vi "Grid_Main.vi"(9 "DC images in":dbl[][][](array[numeric]), 10 "Part of multigrid":bool, 11 "Settings":T3={"Drift Correction Settings"={"Drift Correction every"=1, "Drift correction Pixels"=256, "Channel index (0-23)"=0, "MaxImagesBack"=2, "Threshold"=2, "Increment"=1, "max applied Drift Correction"=20, "Correct Drift"=TRUE, "Correlate"=0, "Correct z drift"=FALSE, "zdrift \nDuration (s)"=0.0}, "Spectroscopy Setting"={"Imaging Current"=5e-12, "ref Current"=5e-12, "tip Speed (m/s)"=2e-09, "Imaging Bias"=0.02, "ref Bias"=0.02, "preSTS delay [ms]"=2000, "STS z offset"=0.0, "during Spec Bias (V)"=0.0015, "trigger1 < Hz"=-6.0, "trigger 2 >Hz"=-4.0, "autoStop"=TRUE, "Spectroscopy"=1, "PLL ON/OFF"=TRUE, "readjust setpoint every "=1, "z Reference (constHeight)"=TRUE, "Lock In"=FALSE}, "Misc"={"File name"="MgPc_perturbed_linezSpec1", "Email when finished"="marina.castelli@monash.edu"}, "Grid Settings"={"type"=0, "type order"=0, "X pixel"=20, "Y pixel"=1, "Grid_Parms"={"center X (m)"=-1.7352741e-07, "center Y (m)"=-2.3765438e-07, "width (m)"=-1.740481e-07, "height (m)"=-2.3958808e-07, "angle (deg)"=-1.0}}} {"Grid Settings"."type order" items=["Grid", "Random", "Adam7"]; "Grid Settings"."type" items=["Line", "Grid", "Cloud"]; "Spectroscopy Setting"."Spectroscopy" items=["Bias", "zSpec"]; "Spectroscopy Setting"."trigger 2 >Hz" format="%#_6p"; "Spectroscopy Setting"."trigger1 < Hz" format="%#_6p"; "Spectroscopy Setting"."during Spec Bias (V)" format="%#_5p"; "Spectroscopy Setting"."STS z offset" format="%#_6p"; "Spectroscopy Setting"."ref Bias" format="%#_6p"; "Spectroscopy Setting"."Imaging Bias" format="%#_6p"; "Spectroscopy Setting"."tip Speed (m/s)" format="%.2p"; "Spectroscopy Setting"."ref Current" format="%#_6p"; "Spectroscopy Setting"."Imaging Current" format="%#_6p"; "Drift Correction Settings"."Correlate" items=["first Frame", "successive Frames"]; "Drift Correction Settings"."max applied Drift Correction" min=1 max=100 step=1 format="%.0p"; "Drift Correction Settings"."Threshold" min=1 step=1; "Drift Correction Settings"."Channel index (0-23)" items=["Current"=0, "Z (m)"=14]}) -> (1 "DC images out":dbl[][][](array[numeric]), 3 "Settings out":T2)   [LabVIEW 2014]
uses:
  <userlib>/Nanonis Prog Interface V5/Nanonis Prog Interface.lvlib
panel:
  in  "resume":T1
  in  "stop":bool
  out "total points":i32=20
  out "Points taken":i32=3
  out "ETA":timestamp=timestamp(3632272774.4134703 s since 1904-01-01)
  out "remaining time":dbl=712.12539879481 format="%<%H:%M:%S>t"
  out "Progress":u8(slide)=15 scale=0.0..100.0 scale format="%#.1g"
  out "Last z adjustment":dbl
  out "Last Drift detected (images back)":i32=1
  out "Y Offset out":sgl=-2.34375e-11 format="%#_6p"
  out "X Offset out":sgl format="%#_6p"
  out "Drift Correction Image":picture
  # "RUN smart tilt before starting the GRID\nCHECK CUTOFF\nmove tip to reference point for tip height"
  # "%"
  # "finish the last action and then"
  # "GRID points"
  # "Increase this if no Drift was detected for \na certain number of images"
  # "% of image size"
  # "Only first frame works"
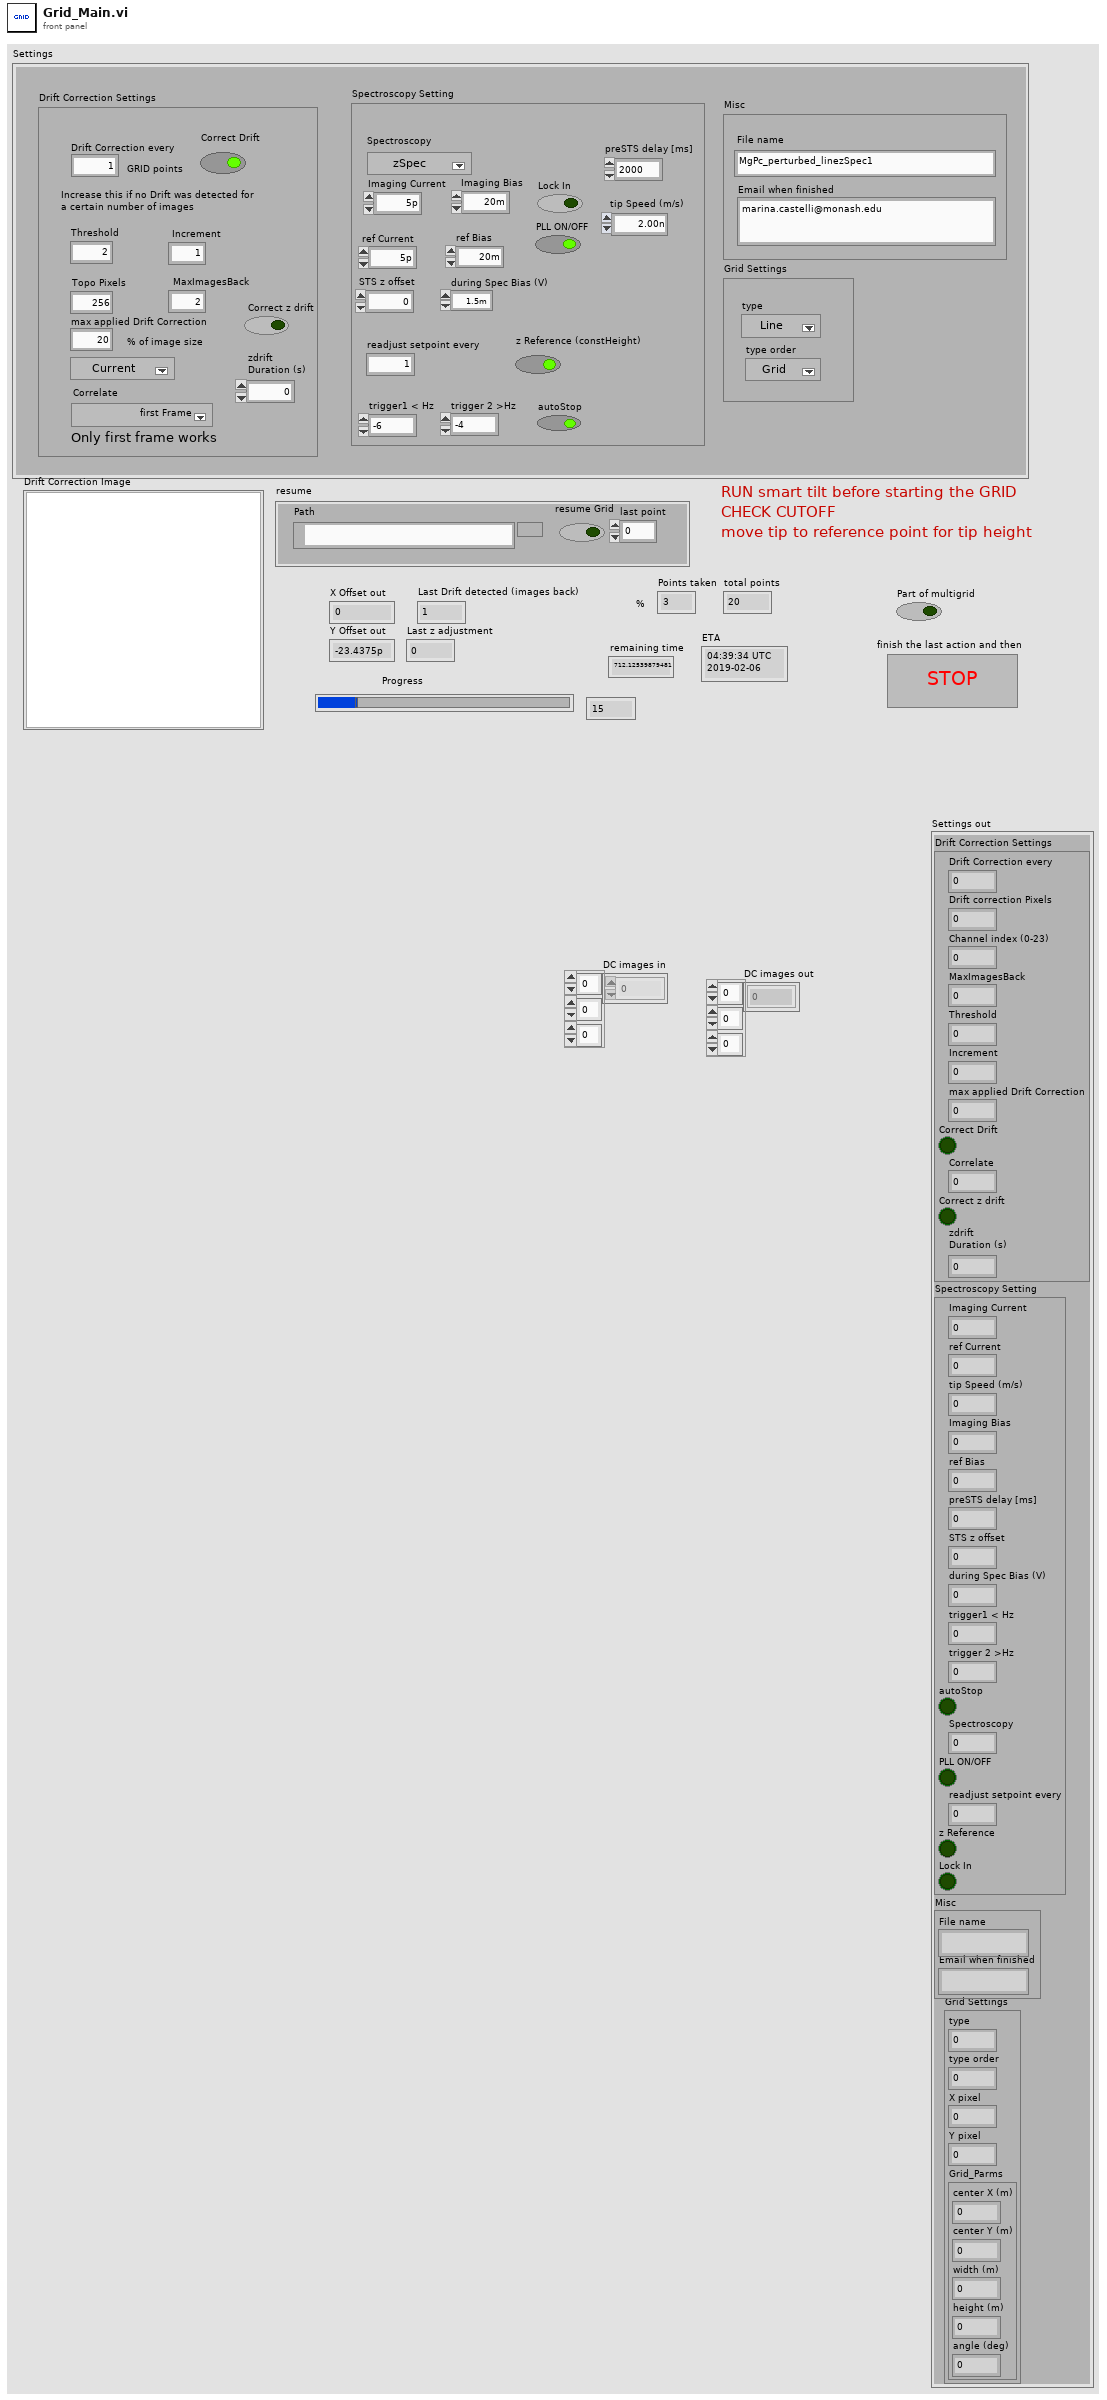
[diagram p1: front panel]
types:
  T1 = cluster{"resume Grid":bool, "Path":path, "last point":i32}
  T2 = cluster{"Drift Correction Settings":cluster{"Drift Correction every":i32, "Drift correction Pixels":i32, "Channel index (0-23)":u8, "MaxImagesBack":i32, "Threshold":i32, "Increment":i32, "max applied Drift Correction":i32, "Correct Drift":bool, "Correlate":u16, "Correct z drift":bool, "zdrift \nDuration (s)":dbl}, "Spectroscopy Setting":cluster{"Imaging Current":dbl, "ref Current":dbl, "tip Speed (m/s)":sgl, "Imaging Bias":dbl, "ref Bias":dbl, "preSTS delay [ms]":u32, "STS z offset":dbl, "during Spec Bias (V)":sgl, "trigger1 < Hz":sgl, "trigger 2 >Hz":sgl, "autoStop":bool, "Spectroscopy":u16, "PLL ON/OFF":bool, "readjust setpoint every ":i32, "z Reference":bool, "Lock In":bool}, "Misc":cluster{"File name":string, "Email when finished":string}, "Grid Settings":cluster{"type":u16, "type order":u16, "X pixel":i32, "Y pixel":i32, "Grid_Parms":cluster{"center X (m)":sgl, "center Y (m)":sgl, "width (m)":sgl, "height (m)":sgl, "angle (deg)":sgl}}}
  T3 = cluster{"Drift Correction Settings":cluster{"Drift Correction every":i32, "Drift correction Pixels":i32, "Channel index (0-23)":u8, "MaxImagesBack":i32, "Threshold":i32, "Increment":i32, "max applied Drift Correction":i32, "Correct Drift":bool, "Correlate":u16, "Correct z drift":bool, "zdrift \nDuration (s)":dbl}, "Spectroscopy Setting":cluster{"Imaging Current":dbl, "ref Current":dbl, "tip Speed (m/s)":sgl, "Imaging Bias":dbl, "ref Bias":dbl, "preSTS delay [ms]":u32, "STS z offset":dbl, "during Spec Bias (V)":sgl, "trigger1 < Hz":sgl, "trigger 2 >Hz":sgl, "autoStop":bool, "Spectroscopy":u16, "PLL ON/OFF":bool, "readjust setpoint every ":i32, "z Reference (constHeight)":bool, "Lock In":bool}, "Misc":cluster{"File name":string, "Email when finished":string}, "Grid Settings":cluster{"type":u16, "type order":u16, "X pixel":i32, "Y pixel":i32, "Grid_Parms":cluster{"center X (m)":sgl, "center Y (m)":sgl, "width (m)":sgl, "height (m)":sgl, "angle (deg)":sgl}}}
  T4 = cluster{"Drift File out":refnum<file>, "zFile":refnum<file>, "BinFile ref":refnum<file>, "xyFile":refnum<file>}
  T5 = cluster{"Drift Correction every":i32, "Drift correction Pixels":i32, "Channel index (0-23)":u8, "MaxImagesBack":i32, "Threshold":i32, "Increment":i32, "max applied Drift Correction":i32, "Correct Drift":bool, "Correlate":u16, "Correct z drift":bool, "zdrift \nDuration (s)":dbl}
  T6 = cluster{"Imaging Current":dbl, "ref Current":dbl, "tip Speed (m/s)":sgl, "Imaging Bias":dbl, "ref Bias":dbl, "preSTS delay [ms]":u32, "STS z offset":dbl, "during Spec Bias (V)":sgl, "trigger1 < Hz":sgl, "trigger 2 >Hz":sgl, "autoStop":bool, "Spectroscopy":u16, "PLL ON/OFF":bool, "readjust setpoint every ":i32, "z Reference":bool, "Lock In":bool}
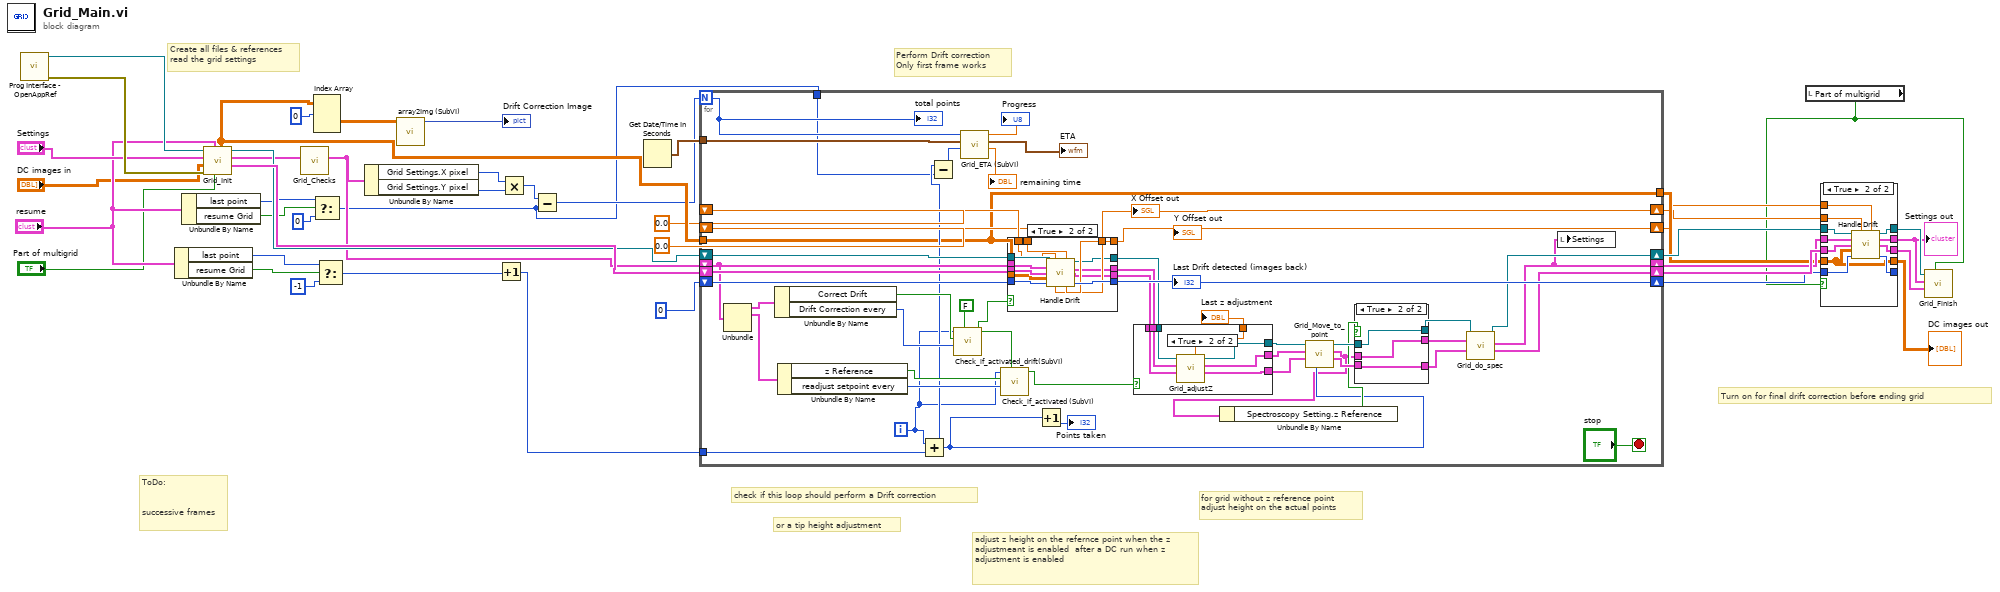
[diagram p0: block diagram]
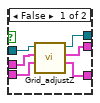
[diagram p3: hidden frame]
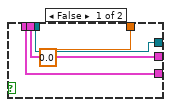
[diagram p4: hidden frame]
diagram:
  # "Turn on for final drift correction before ending grid"
  # "ToDo:\n\n\nsuccessive frames"
  # "Perform Drift correction\nOnly first frame works"
  # "check if this loop should perform a Drift correction"
  # "for grid without z reference point \nadjust height on the actual points"
  # "or a tip height adjustment"
  # "Create all files & references\nread the grid settings"
  # "adjust z height on the refernce point when the z adjustmeant is enabled  after a DC run when z adjustment is enabled"
  n1 = call <userlib>:"Prog Interface - OpenAppRef.vi"() -> ("Error out"=w42:errorcluster, "Application reference"=w43:refnum<vi>)  [unwired: 6 in]
  n2 = Unbundle By Name("resume") -> ("last point"=w24:i32, "resume Grid"=w26:bool)
  n3 = Unbundle By Name("resume") -> ("last point"=w18:i32, "resume Grid"=w20:bool)
  n4 = call "Grid_Init.vi"("Part of multigrid"="Part of multigrid", "resume"="resume", "Error in"=w42, "DC images in"="DC images in", "Settings"="Settings", "Application reference"=w43) -> ("FileRefs"=w40:T4, "Settings out"=w29:T2, "Application ref out"=w39:refnum<vi>, "DC images out"=w37:dbl[][][])  [unwired: 1 in, 1 out]
  n5 = call "Grid_Checks.vi"("Settings"=w29) -> ("Settings out"=w28:T2)  [unwired: 10 in]
  n6 = Index Array(array=w37, index (dim 0)=0 ("index (page)")) -> (element=w38:dbl[][])  [unwired: 2 in]
  n7 = Select(t=w18, s=w20, f=0) -> (s? t:f=w15:i32)
  n8 = Select(t=w24, s=w26, f=-1) -> (s? t:f=w23:i32)
  n9 = Unbundle By Name(w28) -> ("Grid Settings.X pixel"=w32:i32, "Grid Settings.Y pixel"=w31:i32)
  n10 = call "array2Img (SubVI).vi"("Rxy"=w38) -> ("new picture"=→"Drift Correction Image":picture)  [unwired: 10 in]
  n11 = Increment(x=w23) -> (x+1=w21:i32)
  n12 = Multiply(x=w32, y=w31) -> (x*y=w16:i32)
  n13 = Subtract(x=w16, y=w15) -> (x-y=w22:i32)
  n14 = Get Date/Time In Seconds() -> (seconds since 1Jan1904=w30:timestamp)
  n15 = for {
    N: w22 -> [w51]
    tunnel: w37 -> [w45]
    shift-right: [w89] -> w10
    shift-left: 0 ("Last Drift out") -> [w88]
    shift-right: [w84] -> w8
    shift-left: sgl 0.0 ("X Offset out") -> [w87]
    shift-right: [w85] -> w7
    shift-left: sgl 0.0 ("Y Offset out") -> [w86]
    tunnel: w30 -> [w75]
    shift-right: [w72] -> w12
    shift-left: w39 -> [w90]
    shift-right: [w47] -> w13
    shift-left: w28 -> [w58]
    shift-right: [w71] -> w14
    shift-left: w40 -> [w91]
    tunnel: w21 -> [w59]
    tunnel: w15 -> [w48]
    tunnel: [w45] -> w9
    i -> [w44]
    stop <- "stop" stop-if-true
    n16 = Unbundle(w58) -> ("Drift Correction Settings"=w57:T5, "Spectroscopy Setting"=w55:T6)  [unwired: 2 out]
    n17 = Unbundle By Name(w57) -> ("Correct Drift"=w56:bool, "Drift Correction every"=w52:i32)
    n18 = Unbundle By Name(w55) -> ("z Reference"=w54:bool, "readjust setpoint every"=w53:i32)
    n19 = Add(x=w44, y=w59) -> (x+y=w49:i32)
    n20 = Subtract(x=w49, y=w48) -> (x-y=w50:i32)
    n21 = call "Check_if_activated_drift(SubVI).vi"("Override"=FALSE, "activate  every  iterations"=w52, "activated?"=w56, "Iteration"=w44) -> ("perform action"=w80:bool)  [unwired: 7 in]
    n22 = call "Grid_ETA (SubVI).vi"("points taken"=w50, "seconds since 1Jan1904"=w75, "points todo"=w51) -> ("Numeric 4"=→"remaining time":dbl, "Time Stamp"=→"ETA":timestamp, "Numeric 3"=→"Progress":dbl)  [unwired: 6 in]
    n23 = call "Check_if_activated (SubVI).vi"("Override"=w80, "activate  every  iterations"=w53, "activated?"=w54, "Iteration"=w44) -> ("perform action"=w81:bool)  [unwired: 7 in]
    n24 = case shown="True" w80 {
      tunnel: w58 -> [w114 w130]
      tunnel: w91 -> [w113 w129]
      tunnel: w90 -> [w112 w128]
      tunnel: w45 -> [_ w127]
      tunnel: [w115 w126] -> w89
      tunnel: w88 -> [w115 w125]
      tunnel: w87 -> [w117 w124]
      tunnel: w86 -> [w116 w123]
      tunnel: [w116 w122] -> w85
      tunnel: [w117 w121] -> w84
      tunnel: [w112 w120] -> w83
      tunnel: [w114 w119] -> w61
      tunnel: [w113 w118] -> w82
      frame False {
      }
      frame True {
        n25 = call "Handle Drift.vi"("Application ref in"=w128, "X Offset in"=w124, "Y Offset In"=w123, "Settings"=w130, "FileRefs"=w129, "Drift Correction image"=w127, "Last Drift"=w125) -> ("Application out"=w120:refnum<vi>, "Settings out"=w119:T2, "FileRefs out File Refs  Out"=w118:T4, "X Offset out"=w121:sgl, "Y Offset out"=w122:sgl, "Last Drift out"=w126:i32)  [unwired: 3 in]
      }
    }
    "X Offset out" <- w84
    "Y Offset out" <- w85
    "Last Drift detected (images back)" <- w89
    n26 = Increment(x=w49) -> (x+1=→"Points taken":i32)
    n27 = case shown="True" w81 {
      tunnel: w83 -> [w103 w111]
      tunnel: w82 -> [w102 w110]
      tunnel: w61 -> [w101 w109]
      tunnel: [w102 w108] -> w74
      tunnel: [w101 w107] -> w63
      tunnel: [w103 w106] -> w73
      tunnel: [0.0 ("Last z adjustment") w105] -> w70
      frame False {
      }
      frame True {
        n28 = call "Grid_adjustZ.vi"("FileRefs"=w110, "Settings"=w109, "Application in"=w111) -> ("FileRefs out"=w108:T4, "Settings out"=w107:T2, "Application ref out"=w106:refnum<vi>, "Last z adjustment"=w105:dbl)  [unwired: 4 in, 1 out]
      }
    }
    "Last z adjustment" <- w70
    n29 = call "Grid_Move_to_point.vi"("point"=w49, "FileRefs in"=w74, "Settings"=w63, "Application ref in"=w73) -> ("FileRefs out"=w65:T4, "Settings out"=w46:T2, "Application ref out"=w66:refnum<vi>)  [unwired: 5 in]
    n30 = Unbundle By Name(w46) -> ("Spectroscopy Setting.z Reference"=w64:bool)
    n31 = case shown="True" w64 {
      tunnel: [w97 w100] -> w69
      tunnel: [w96 w98] -> w67
      tunnel: [w95 w99] -> w68
      tunnel: w66 -> [w94 w100]
      tunnel: w46 -> [w93 w99]
      tunnel: w65 -> [w92 w98]
      frame False {
        n32 = call "Grid_adjustZ.vi"("FileRefs"=w92, "Settings"=w93, "Application in"=w94) -> ("FileRefs out"=w96:T4, "Settings out"=w95:T2, "Application ref out"=w97:refnum<vi>)  [unwired: 4 in, 2 out]
      }
      frame True {
      }
    }
    n33 = call "Grid_do_spec.vi"("FileRefs in"=w67, "Settings in"=w68, "Application ref in"=w69) -> ("FileRefs out"=w71:T4, "Settings out"=w47:T2, "Application ref out"=w72:refnum<vi>)  [unwired: 5 in, 1 out]
    n34 = local write "Settings"(w47) -> ()
    "total points" <- w51
  }
  n35 = local read "Part of multigrid"() -> (w4:bool)
  n36 = case shown="True" w4 {
    tunnel: w13 -> [w134 w146]
    tunnel: w14 -> [w133 w145]
    tunnel: w12 -> [w132 w144]
    tunnel: [w135 w143] -> _
    tunnel: w10 -> [w135 w139]
    tunnel: [w132 w142] -> w11
    tunnel: [w134 w141] -> w5
    tunnel: [w133 w140] -> w6
    tunnel: w9 -> [w131 w136]
    tunnel: w8 -> [_ w138]
    tunnel: w7 -> [_ w137]
    tunnel: [w131 w136] -> w2
    frame False {
    }
    frame True {
      n37 = call "Handle Drift.vi"("Application ref in"=w144, "X Offset in"=w138, "Y Offset In"=w137, "Settings"=w146, "FileRefs"=w145, "Drift Correction image"=w136, "Last Drift"=w139) -> ("Application out"=w142:refnum<vi>, "Settings out"=w141:T2, "FileRefs out File Refs  Out"=w140:T4, "Last Drift out"=w143:i32)  [unwired: 3 in, 2 out]
    }
  }
  "Settings out" <- w5
  "DC images out" <- w2
  n38 = call "Grid_Finish.vi"("Part of multigrid"=w4, "FileRefs"=w6, "Settings"=w5, "Application reference"=w11) -> ()  [unwired: 8 in]
